vi "RSZVB Set Calibration Power Offset.vi"(7 "Calibration Power Offset (0)":dbl format="%^.3e", 8 "error in (no error)":errorcluster {"code" format="%.0x"}, 9 "Port Number (1)":i32=1, 10 "Channel (1)":i32=1, 11 "VISA session":refnum<visa-resource-name>) -> (0 "error out":errorcluster {"code" format="%.0x"}, 3 "dup VISA session":refnum<visa-resource-name>)   [LabVIEW 2011]
doc: "This VI specifies a gain (positive values) or an attenuation (negative values) in the signal path between the source port and the calibrated reference plane. The value has no impact on the source power. \n\nRemote-control command(s):\nSOURce<Ch>:POWer<Pt>:CORRection:LEVel:OFFSet <numeric_value>"
uses:
  _utility/RSZVB Global Data.vi
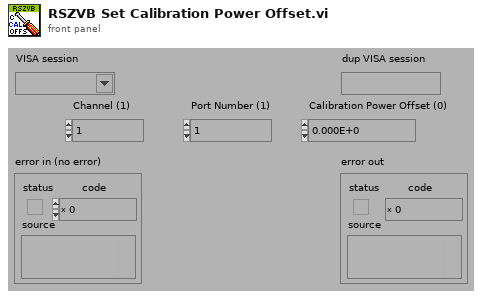
[diagram p1: front panel]
types:
  T1 = cluster{"Error Checking (T: On)":bool, "Installed Options":string[], "Data Valid?":bool, "Ports":i32, "Model":string[], "Option Checking (T: On)":bool}[]
  T2 = cluster{"Error Checking (T: On)":bool, "Installed Options":string[], "Data Valid?":bool, "Ports":i32, "Model":string[], "Option Checking (T: On)":bool}
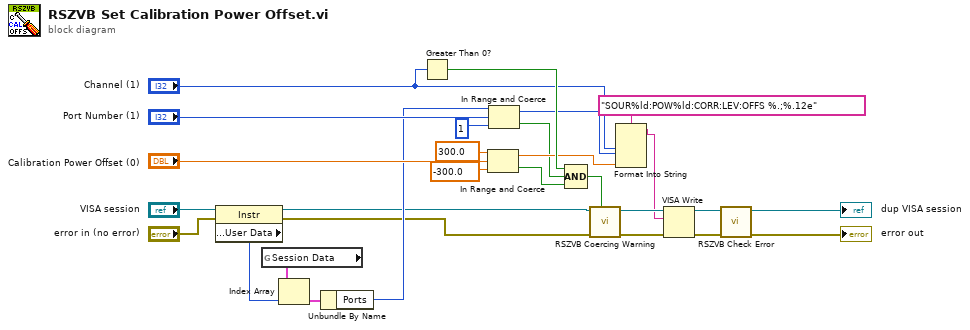
[diagram p0: block diagram]
diagram:
  n1 = property class="Instr"(reference="VISA session", error in="error in (no error)") -> (reference out=w6:refnum<visa-resource-name>, error out=w5:errorcluster, "General Settings:User Data"=w12:u32)
  n2 = global read "RSZVB Global Data.vi" "Session Data"() -> (w13:T1)
  n3 = Index Array(array=w13, index=w12) -> (element=w14:T2)
  n4 = Unbundle By Name(w14) -> ("Ports"=w9:i32)
  n5 = Greater Than 0?(x="Channel (1)") -> (x > 0?=w20:bool)
  n6 = In Range and Coerce(upper limit=300.0, x="Calibration Power Offset (0)", lower limit=-300.0) -> (coerced(x)=w3:dbl, In Range?=w2:bool)
  n7 = In Range and Coerce(upper limit=w9, x="Port Number (1)", lower limit=1) -> (coerced(x)=w4:i32, In Range?=w1:bool)
  n8 = Compound Arithmetic op=AND(w20, w1, w2) -> (w19:bool)
  n9 = call "RSZVB Coercing Warning.vi"("In Range?"=w19, "error in (no error)"=w5, "VISA session"=w6) -> ("error out"=w27:errorcluster, "dup VISA session"=w28:refnum<visa-resource-name>)  [unwired: 7 in]
  n10 = Format Into String(format string="SOUR%ld:POW%ld:CORR:LEV:OFFS %.;%.12e", "Channel (1)", w4, w3) -> (resulting string=w23:string)  [unwired: 2 in, 1 out]
  n11 = VISA Write(VISA resource name=w28, write buffer=w23, error in (no error)=w27) -> (VISA resource name out=w25:refnum<visa-resource-name>, error out=w26:errorcluster)  [unwired: 1 out]
  n12 = call "RSZVB Check Error.vi"("error in (no error)"=w26, "VISA session"=w25) -> ("error out"=→"error out":errorcluster, "dup VISA session"=→"dup VISA session":refnum<visa-resource-name>)  [unwired: 8 in]
